vi "Delete Multiple Frames.vi"(8 "error in (no error)":errorcluster, 11 "Node Ptr":u64 format="%.0x") -> (0 "error out":errorcluster)   [LabVIEW 2020, in "FlexRay Custom Device System Explorer.lvlib"]
uses:
  FlexRay Custom Device System Explorer.lvlib
  <vilib>/Utility/error.llb/DialogType.ctl
  <vilib>/NI VeriStand/Custom Device API/Custom Device Item Ref.ctl
  <vilib>/NI VeriStand/Custom Device API/Custom Device API.lvlib
panel:
  in  "Frames":i32[](listbox)
  in  "Cancel":bool
  in  "Apply":bool
  in  "Tag":string
  # "Use ctrl or shift to select multiple frames"
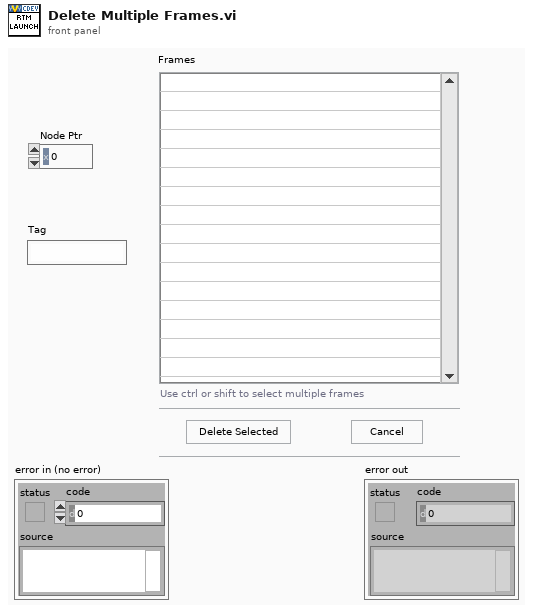
[diagram p1: front panel]
types:
  T1 = typedef "Custom Device API.lvlib/Custom Device Item Ref.ctl" = u64
  T2 = enum16{"Init", "WaitOnUserInput", "Action", "Cleanup"}
  T3 = typedef "DialogType.ctl" = u16
  T4 = typedef "Custom Device API.lvlib/Custom Device Item Info.ctl" = cluster{"Name":string, "Is Channel":bool, "GUID":string, "Is Waveform":bool}
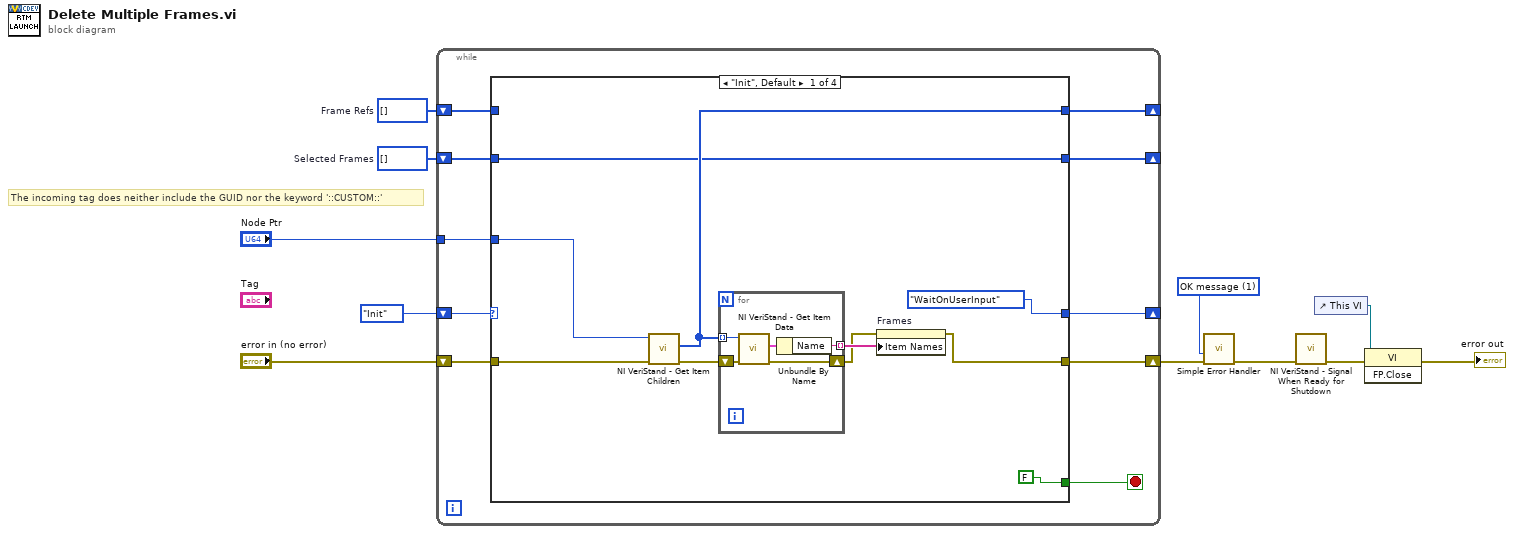
[diagram p0: block diagram]
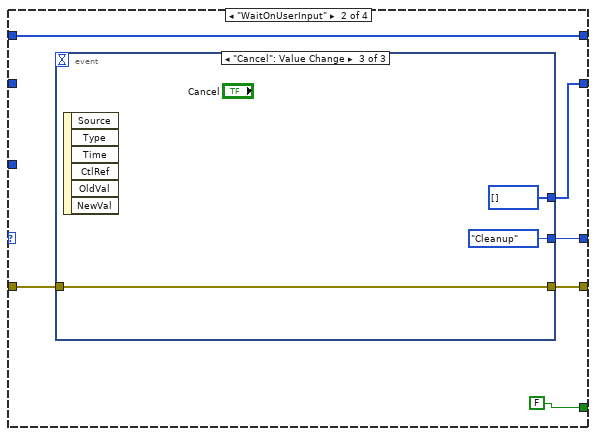
[diagram p2: hidden frame]
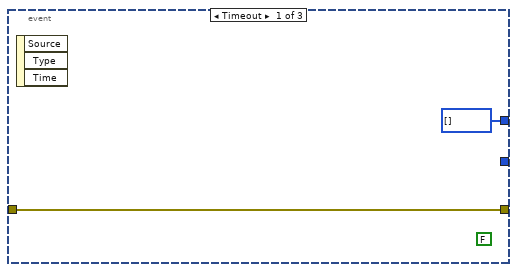
[diagram p3: hidden frame]
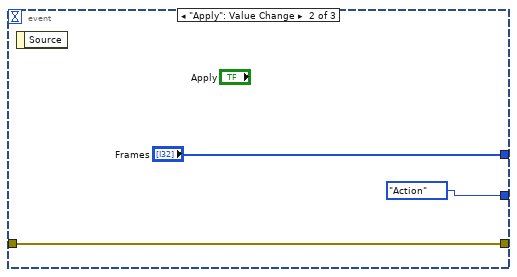
[diagram p4: hidden frame]
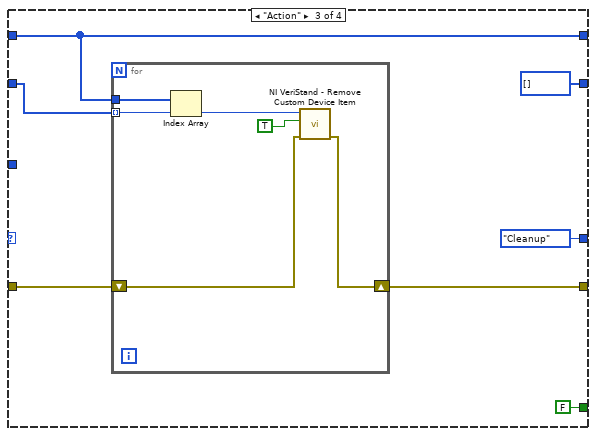
[diagram p5: hidden frame]
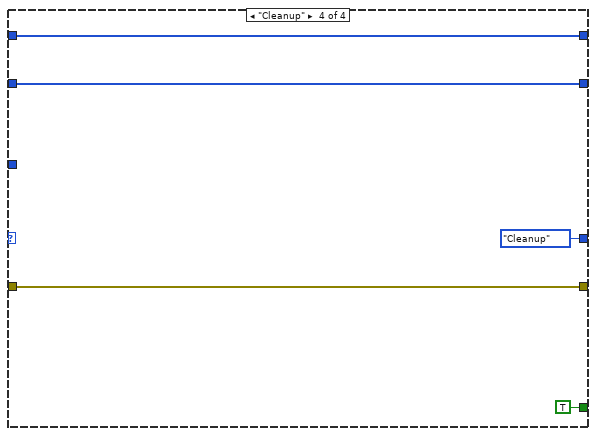
[diagram p6: hidden frame]
diagram:
  w2 = i32[] []  # Selected Frames
  w3 = T1[] []  # Frame Refs
  w8 = T3 1 items=["no dialog", "OK message", "continue or stop message", "OK message + warnings", "continue/stop + warnings"] ("type of dialog (OK msg:1)")
  # "The incoming tag does neither include the GUID nor the keyword '::CUSTOM::'"
  n1 = while {
    tunnel: "Node Ptr" -> [w18]
    shift-right: [w17] -> w1
    shift-left: "error in (no error)" -> [w19]
    shift-right: [w16] -> _
    shift-left: w3 -> [w15]
    shift-right: [w21] -> _
    shift-left: w2 -> [w13]
    shift-right: [w12] -> _
    shift-left: T2."Init" -> [w20]
    stop <- w14 stop-if-true
    n2 = case shown="\"Init\", Default" w20 {
      tunnel: [w22 w42 i32[] [] ("Frames") w67] -> w21
      tunnel: w19 -> [w30 w40 w54 w66]
      tunnel: w18 -> [w29 _ _ _]
      tunnel: [w27 w41 w53 w66] -> w17
      tunnel: [w26 w38 w57 w68] -> w16
      tunnel: w15 -> [_ w38 w57 w68]
      tunnel: [FALSE FALSE FALSE TRUE] -> w14
      tunnel: w13 -> [w22 _ w55 w67]
      tunnel: [T2."WaitOnUserInput" w37 T2."Cleanup" T2."Cleanup"] -> w12
      frame "Init", Default {
        n3 = call <vilib>:"NI VeriStand - Get Item Children.vi"("error in (no error)"=w30, "Item Ref in"=w29) -> ("error out"=w25:errorcluster, "Child Refs"=w26:T1[])  [unwired: 6 in, 2 out]
        n4 = for {
          tunnel: w26 -> [w36] mode=indexing
          tunnel: [w34] -> w31 mode=indexing
          shift-right: [w33] -> w28
          shift-left: w25 -> [w32]
          n5 = call <vilib>:"NI VeriStand - Get Item Data.vi"("error in (no error)"=w32, "Item Ref in"=w36) -> ("error out"=w33:errorcluster, "Item Info"=w35:T4)  [unwired: 6 in, 2 out]
          n6 = Unbundle By Name(w35) -> ("Name"=w34:string)
        }
        n7 = property on="Frames" class="LstBox (strict)"(error in=w28, "Item Names"=w31) -> (error out=w27:errorcluster)  [unwired: 1 in, 1 out]
      }
      frame "WaitOnUserInput" {
        n8 = event shown="[2] \"Cancel\": Value Change" {
          selector: _ -> [_ _ _]
          dyn-events: _ -> [_ _ _]
          timeout: _ -> [_ _ _]
          tunnel: [i32[] [] ("Frames") "Frames" i32[] [] ("Frames")] -> w42
          tunnel: [w43 w45 w49] -> w41
          tunnel: w40 -> [w43 w45 w49]
          tunnel: [_ T2."Action" T2."Cleanup"] -> w37
          event Timeout {
            (unwired) FALSE
            n9 = event-data() -> ()  [unwired: 1 in, 3 out]
          }
          event "Apply": Value Change {
            n10 = event-data() -> ()  [unwired: 1 in, 1 out]
          }
          event "Cancel": Value Change {
            n11 = event-data() -> ()  [unwired: 1 in, 6 out]
          }
        }
      }
      frame "Action" {
        n12 = for {
          tunnel: w57 -> [w63]
          tunnel: w55 -> [w62] mode=indexing
          shift-right: [w58] -> w53
          shift-left: w54 -> [w59]
          n13 = Index Array(array=w63, index=w62) -> (element=w61:T1)
          n14 = call <vilib>:"NI VeriStand - Remove Custom Device Item.vi"("error in (no error)"=w59, "Force Delete (F)"=TRUE, "Item Ref in"=w61) -> ("error out"=w58:errorcluster)  [unwired: 7 in, 1 out]
        }
      }
      frame "Cleanup" {
      }
    }
  }
  n15 = call <vilib>:"Simple Error Handler.vi"("type of dialog (OK msg:1)"=w8, "error in (no error)"=w1) -> ("error out"=w9:errorcluster)  [unwired: 3 in, 4 out]
  n16 = call <vilib>:"NI VeriStand - Signal When Ready for Shutdown.vi"("error in (no error)"=w9) -> ("error out"=w11:errorcluster)  [unwired: 10 in]
  n17 = control-ref of="This VI"() -> (w10:refnum<vi>)
  n18 = invoke class="VI" method="FP.Close"(reference=w10, error in=w11) -> (error out=→"error out":errorcluster)  [unwired: 1 in, 2 out]
